vi "Set Message Trigger.vi"(7 "nodeID":T1 format="%.0x", 8 "error in (no error)":errorcluster, 11 "Trigger Channel in":T1 format="%.0x") -> (0 "error out":errorcluster, 3 "Trigger Channel out":T1 format="%.0x")   [LabVIEW 2023, in "Instrument Addon Scripting API.lvlib"]
uses:
  Instrument Addon Scripting API.lvlib
  <vilib>/NI VeriStand/Custom Device API/Custom Device Item Ref.ctl
  Addon/Addon Shared/Types/FG Control.ctl
  Addon/Addon Shared/SubVIs/Constants.vi
  <vilib>/NI VeriStand/Custom Device API/NI VeriStand - Get Item Property.vi
  <vilib>/NI VeriStand/Custom Device API/Get Item Property (Boolean).vi
  <vilib>/NI VeriStand/Custom Device API/Get Item Property (String).vi
  <vilib>/NI VeriStand/Custom Device API/NI VeriStand - Set Item Property.vi
  <vilib>/NI VeriStand/Custom Device API/Set Item Property (Boolean).vi
  <vilib>/NI VeriStand/Custom Device API/Set Item Property (String).vi
  NationalInstruments.VeriStand.SystemStorage
  Addon/Addon Shared/Instrument Addon Shared.lvlib
  <vilib>/NI VeriStand/Custom Device API/Custom Device API.lvlib
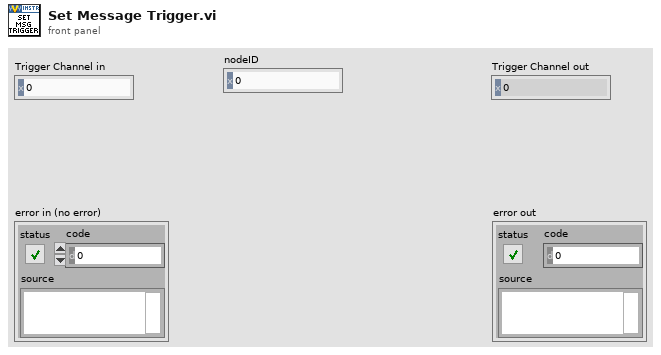
[diagram p1: front panel]
types:
  T1 = typedef "Custom Device API.lvlib/Custom Device Item Ref.ctl" = u64
  T2 = typedef "Instrument Addon Shared.lvlib/FG Control.ctl" = enum16{"Get", "Set"}
  T3 = typedef "Instrument Addon Shared.lvlib/Trigger Parameters.ctl" = cluster{"Use Channel":bool, "Channel Path":string}
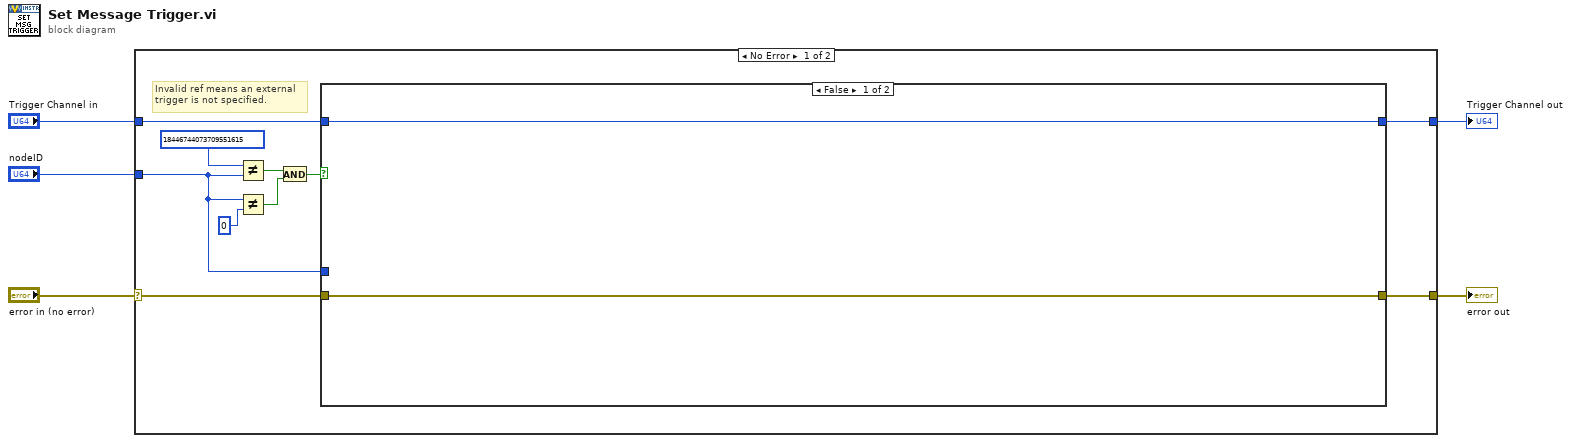
[diagram p0: block diagram]
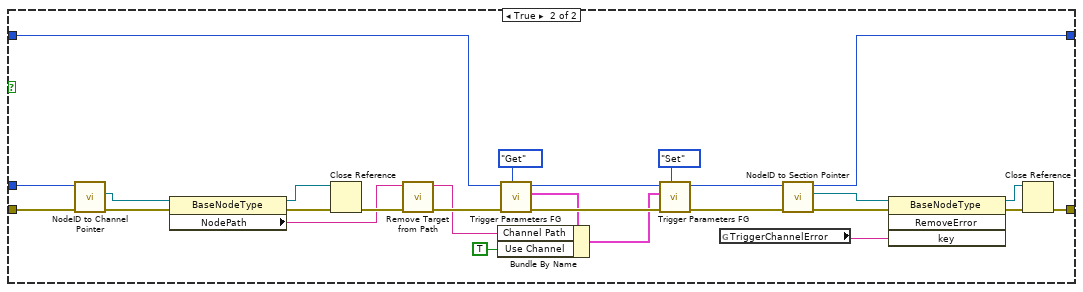
[diagram p2: hidden frame]
diagram:
  n1 = case shown="No Error" "error in (no error)" {
    selector: "error in (no error)" -> [w11 w46]
    tunnel: "Trigger Channel in" -> [w15 w45]
    tunnel: [w14 w46] -> w4
    tunnel: [w13 w45] -> w3
    tunnel: "nodeID" -> [w10 _]
    frame No Error {
      # "Invalid ref means an external\ntrigger is not specified."
      n2 = Not Equal?(x=T1 18446744073709551615, y=w10) -> (x != y?=w8:bool)
      n3 = Not Equal?(x=w10, y=T1 0 ("x")) -> (x != y?=w7:bool)
      n4 = And(x=w8, y=w7) -> (x .and. y?=w6:bool)
      n5 = case shown="False" w6 {
        tunnel: w15 -> [w17 w35]
        tunnel: [w16 w34] -> w14
        tunnel: w11 -> [w16 w25]
        tunnel: w10 -> [_ w23]
        tunnel: [w17 w27] -> w13
        frame False {
        }
        frame True {
          n6 = call "NodeID to Channel Pointer.vi"("error in (no error)"=w25, "nodeID in"=w23) -> ("error out"=w24:errorcluster, "BaseNodeType out"=w22:refnum<k24>)  [unwired: 7 in, 1 out]
          n7 = property class="BaseNodeType"(reference=w22, error in=w24) -> (reference out=w32:refnum<k24>, error out=w33:errorcluster, "NodePath"=w19:string)
          n8 = Close Reference(reference=w32, error in (no error)=w33) -> (error out=w21:errorcluster)
          n9 = call "Remove Target from Path.vi"("error in (no error)"=w21, "NodePath"=w19) -> ("error out"=w20:errorcluster, "PathArrayToString"=w18:string)  [unwired: 8 in]
          n10 = call "Trigger Parameters FG.vi"("Action"=FG_Control."Get", "error in (no error)"=w20, "Item Ref in"=w35) -> ("error out"=w41:errorcluster, "Trigger Parameters"=w39:T3, "Item Ref out"=w40:T1)  [unwired: 6 in]
          n11 = Bundle By Name(cluster=w39, "Channel Path"=w18, "Use Channel"=TRUE) -> (w36:T3)
          n12 = call "Trigger Parameters FG.vi"("Action"=FG_Control."Set", "error in (no error)"=w41, "Trigger Parameters"=w36, "Item Ref in"=w40) -> ("error out"=w29:errorcluster, "Item Ref out"=w28:T1)  [unwired: 5 in, 1 out]
          n13 = global read "Constants.vi" "TriggerChannelError"() -> (w44:string)
          n14 = call "NodeID to Section Pointer.vi"("error in (no error)"=w29, "nodeID in"=w28) -> ("error out"=w30:errorcluster, "BaseNodeType out"=w26:refnum<k24>, "nodeID out"=w27:T1)  [unwired: 7 in]
          n15 = invoke class="BaseNodeType" method="RemoveError"(reference=w26, error in=w30, "key"=w44) -> (reference out=w42:refnum<k24>, error out=w43:errorcluster)  [unwired: 1 in, 2 out]
          n16 = Close Reference(reference=w42, error in (no error)=w43) -> (error out=w34:errorcluster)
        }
      }
    }
    frame Error {
    }
  }
  "Trigger Channel out" <- w3
  "error out" <- w4
